vi "Generic Error Response.vi"(6 "Include Message?":bool, 8 "error in (no error)":errorcluster) -> (0 "error out":errorcluster, 3 "Response out":refnum<class "Response.lvclass">)   [LabVIEW 2020, in "HTTP Server.lvlib" / "Server.lvclass"]
uses:
  Server.lvclass
  lv-http-util/HTTP Utils/Response/Response.lvclass
  <vilib>/Utility/error.llb/DialogType.ctl
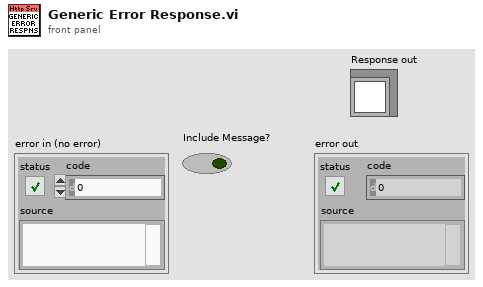
[diagram p1: front panel]
types:
  T1 = typedef "DialogType.ctl" = u16
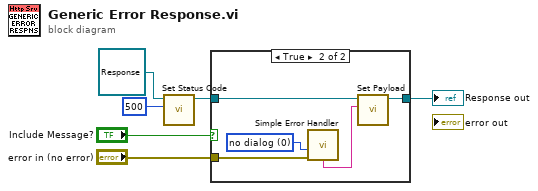
[diagram p0: block diagram]
diagram:
  n1 = call "Set Status Code.vi"("Status Code"=u16 500, "Response in"=refnum<class "Response.lvclass"> refnum) -> ("Response out"=w3:refnum<class "Response.lvclass">)  [unwired: 8 in, 1 out]
  n2 = case shown="True" "Include Message?" {
    tunnel: w3 -> [w7 w12]
    tunnel: "error in (no error)" -> [_ w10]
    tunnel: [w7 w11] -> w1
    frame False {
    }
    frame True {
      w9 = T1 0 items=["no dialog", "OK message", "continue or stop message", "OK message + warnings", "continue/stop + warnings"] ("type of dialog (OK msg:1)")
      n3 = call <vilib>:"Simple Error Handler.vi"("type of dialog (OK msg:1)"=w9, "error in (no error)"=w10) -> ("message"=w8:string)  [unwired: 3 in, 4 out]
      n4 = call "Set Payload.vi"("Payload"=w8, "Response in"=w12) -> ("Response out"=w11:refnum<class "Response.lvclass">)  [unwired: 8 in, 1 out]
    }
  }
  "Response out" <- w1
